vi "read scanivalve config file.vi"(11 "scanivalve config file":path=path "\\\\Mac\\Home/OneDrive - Imperial College London/LabVIEW/Compressor Rig V2/RT/Data processor/scanivalve config.csv") -> (3 "output array":T1[][](array[typedef]))   [LabVIEW 2018]
uses:
  type defs/scanivalve channel control.ctl
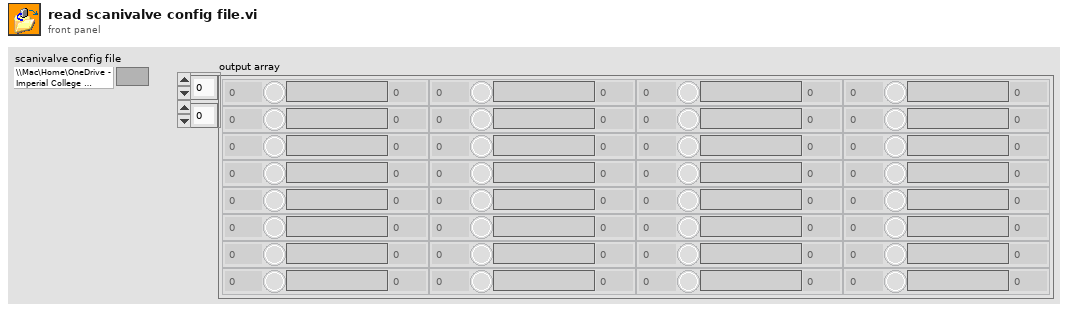
[diagram p1: front panel]
types:
  T1 = typedef "scanivalve channel control.ctl" = cluster{"port":u16, "active":bool, "channelName":string, "range":dbl}
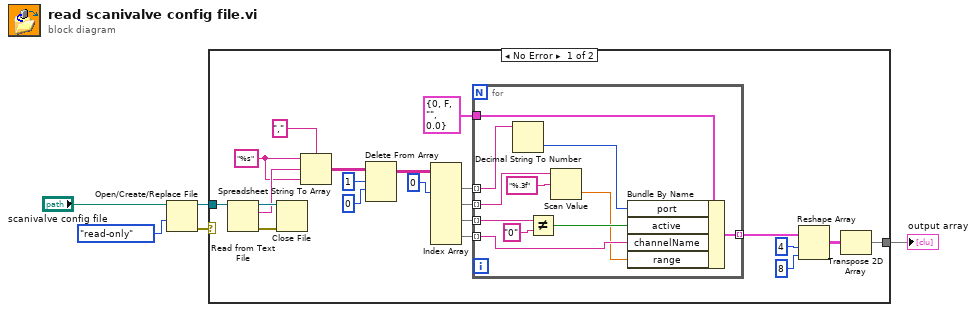
[diagram p0: block diagram]
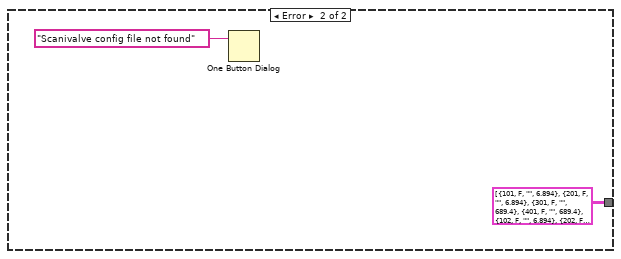
[diagram p2: hidden frame]
diagram:
  n1 = Open/Create/Replace File(file path (use dialog)="scanivalve config file", access (0:read/write)=enum16{"read/write", "read-only", "write-only"}."read-only") -> (refnum out=w4:refnum<file>, error out=w1:errorcluster)  [unwired: 4 in, 1 out]
  n2 = case shown="No Error" w1 {
    tunnel: w4 -> [w26 _]
    tunnel: [w10 T1[][] [[{"port"=101, "active"=FALSE, "channelName"="", "range"=6.894}, {"port"=201, "active"=FALSE, "channelName"="", "range"=6.894}, {"port"=301, "active"=FALSE, "channelName"="", "range"=689.4}, {"port"=401, "active"=FALSE, "channelName"="", "range"=689.4}], [{"port"=102, "active"=FALSE, "channelName"="", "range"=6.894}, {"port"=202, "active"=FALSE, "channelName"="", "range"=6.894}, {"port"=302, "active"=FALSE, "channelName"="", "range"=689.4}, {"port"=402, "active"=FALSE, "channelName"="", "range"=689.4}], [{"port"=103, "active"=FALSE, "channelName"="", "range"=6.894}, {"port"=203, "active"=FALSE, "channelName"="", "range"=6.894}, {"port"=303, "active"=FALSE, "channelName"="", "range"=689.4}, {"port"=403, "active"=FALSE, "channelName"="", "range"=689.4}], [{"port"=104, "active"=FALSE, "channelName"="", "range"=6.894}, {"port"=204, "active"=FALSE, "channelName"="", "range"=6.894}, {"port"=304, "active"=FALSE, "channelName"="", "range"=689.4}, {"port"=404, "active"=FALSE, "channelName"="", "range"=689.4}], [{"port"=109, "active"=FALSE, "channelName"="", "range"=6.894}, {"port"=209, "active"=FALSE, "channelName"="", "range"=6.894}, {"port"=309, "active"=FALSE, "channelName"="", "range"=689.4}, {"port"=409, "active"=FALSE, "channelName"="", "range"=689.4}], [{"port"=110, "active"=FALSE, "channelName"="", "range"=6.894}, {"port"=210, "active"=FALSE, "channelName"="", "range"=6.894}, {"port"=310, "active"=FALSE, "channelName"="", "range"=689.4}, {"port"=410, "active"=FALSE, "channelName"="", "range"=689.4}], [{"port"=111, "active"=FALSE, "channelName"="", "range"=6.894}, {"port"=211, "active"=FALSE, "channelName"="", "range"=6.894}, {"port"=311, "active"=FALSE, "channelName"="", "range"=689.4}, {"port"=411, "active"=FALSE, "channelName"="", "range"=689.4}], [{"port"=112, "active"=FALSE, "channelName"="", "range"=6.894}, {"port"=212, "active"=FALSE, "channelName"="", "range"=6.894}, {"port"=312, "active"=FALSE, "channelName"="", "range"=689.4}, {"port"=412, "active"=FALSE, "channelName"="", "range"=689.4}]] ("output array 2")] -> w2
    frame No Error {
      w22 = "%s" ("format string")
      n3 = Read from Text File(file (use dialog)=w26) -> (refnum out=w24:refnum<file>, text=w23:string, error out=w25:errorcluster)  [unwired: 3 in, 1 out]
      n4 = Close File(refnum=w24, error in=w25) -> ()  [unwired: 2 out]
      n5 = Spreadsheet String To Array(delimiter (Tab)=",", format string=w22, spreadsheet string=w23, array type (2D Dbl)=w22) -> (array=w9:string[][])
      n6 = Delete From Array(array=w9, length=1, index (row)=0) -> (array with subset deleted=w6:string[][])  [unwired: 1 in, 1 out]
      n7 = Index Array(array=w6, index (col) #1=0 ("disabled index (col)")) -> (element #1=w19:string[], element #2=w18:string[], element #3=w17:string[], element #4=w15:string[])  [unwired: 7 in]
      n8 = for {
        tunnel: w19 -> [w37] mode=indexing
        tunnel: w18 -> [w36] mode=indexing
        tunnel: w17 -> [w34] mode=indexing
        tunnel: T1 {"port"=0, "active"=FALSE, "channelName"="", "range"=0.0} ("scanivalveChannel") -> [w32]
        tunnel: w15 -> [w29] mode=indexing
        tunnel: [w27] -> w14 mode=indexing
        n9 = Decimal String To Number(string=w37) -> (number=w31:i32)  [unwired: 2 in, 1 out]
        n10 = Not Equal?(x=w34, y="0") -> (x != y?=w30:bool)
        n11 = Scan Value(string=w36, format string="%.3f") -> (value=w28:dbl)  [unwired: 1 in, 1 out]
        n12 = Bundle By Name(cluster=w32, "port"=w31, "active"=w30, "channelName"=w29, "range"=w28) -> (w27:T1)
      }
      n13 = Reshape Array(w14, 4 ("dimension size"), 8 ("dimension size")) -> (w11:T1[][])
      n14 = Transpose 2D Array(2D array=w11) -> (transposed array=w10:T1[][])
    }
    frame Error {
      n15 = One Button Dialog(message="Scanivalve config file not found") -> ()  [unwired: 1 in, 1 out]
    }
  }
  "output array" <- w2
